vi "Write Multiple Registers.vi"(8 "error in":errorcluster, 9 "register values":u16[](array[numeric]), 10 "starting address":u16, 11 "device data model in":refnum<class "Standard Data Model.lvclass">) -> (0 "error out":errorcluster, 3 "device data model out":refnum<class "Standard Data Model.lvclass">)   [LabVIEW 2021, in "Standard Data Model.lvclass"]
doc: "Writes the values of multiple register values in series, starting at address M."
uses:
  Standard Data Model.lvclass
  Standard Data Model.lvclass/Standard Data Model.ctl
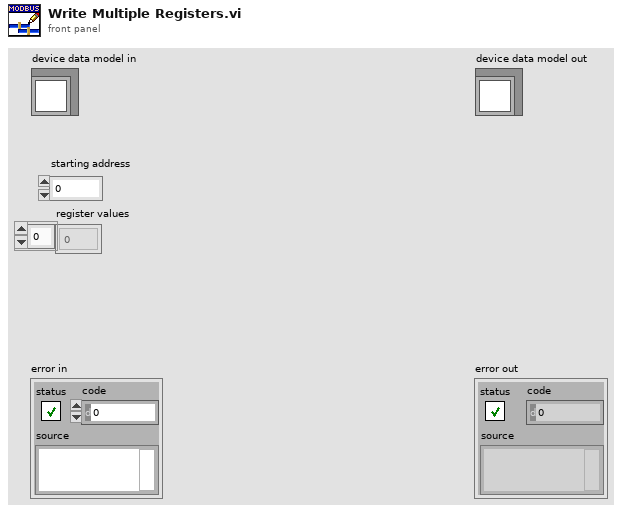
[diagram p1: front panel]
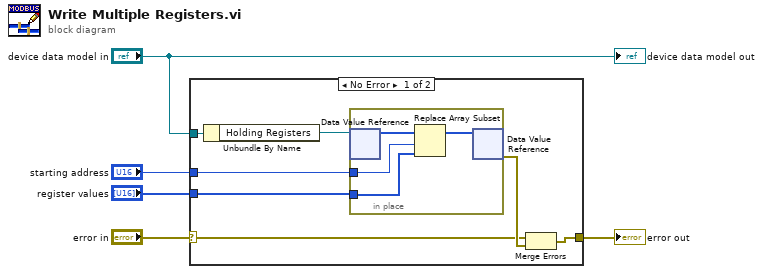
[diagram p0: block diagram]
diagram:
  n1 = case shown="No Error" "error in" {
    selector: "error in" -> [w6 w17]
    tunnel: "device data model in" -> [w12 _]
    tunnel: [w11 w17] -> w4
    tunnel: "register values" -> [w8 _]
    tunnel: "starting address" -> [w7 _]
    frame No Error {
      n2 = Unbundle By Name(w12) -> ("Holding Registers"=w9:refnum<data-value>)
      n3 = in-place {
        in-place-border: w8 -> [w16]
        in-place-border: w7 -> [w15]
        n4 = in-place-dvr #1(w9) -> (w14:u16[])  [unwired: 1 out]
        n5 = Replace Array Subset(array=w14, new element=w16, index=w15) -> (w13:u16[])
        n6 = in-place-dvr #1(w13) -> (w10:errorcluster)  [unwired: 1 out]
      }
      n7 = Merge Errors(w6, w10) -> (w11:errorcluster)
    }
    frame Error {
    }
  }
  "error out" <- w4
  "device data model out" <- "device data model in"
